vi "Algae Teleop Handler.vi"() -> ()   [LabVIEW 2023]
uses:
  Teleop Util/Algae States.ctl
  <vilib>/Rock Robotics/WPI/Joystick/XBox Buttons Indexer.ctl
  <vilib>/Rock Robotics/WPI/Joystick/XBox Axes Indexer.ctl
  Algae/Implementation/Algae Operations.ctl
  918af4a3-8dae-4537-8dc6-29252aaed449.vi
  <vilib>/Rock Robotics/WPI/Utilities/WPI_GetSetVariantRefNum.vi
  Framework/Robot Global Data.vi
panel:
  in  "Setpoint":dbl
  out "s? t:f":T1=enum."Intake Algae"
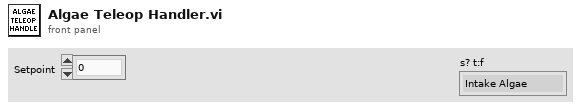
[diagram p1: front panel]
types:
  T1 = typedef "Algae States.ctl" = enum16{"Idle", "Intake Algae", "Outtake Algae", "Stow", "Manual Overrides"}
  T2 = typedef "XBox Axes Indexer.ctl" = enum16{"Left X", "Left Y", "Left Trigger", "Right Trigger", "Right X", "Right Y"}
  T3 = typedef "XBox Buttons Indexer.ctl" = enum16{"A", "B", "X", "Y", "Left Bumper", "Right Bumper", "Back", "Start", "Left Joystick", "Right Joystick"}
  T4 = typedef "WPI_JoystickDevRef.ctl" = cluster{"Device":T5}
  T5 = typedef "WPI_JoystickDeviceEnum.ctl" = enum16{"USB 0", "USB 1", "USB 2", "USB 3", "USB 4", "USB 5"}
  T6 = typedef "Algae Operations.ctl" = enum16{"Reserve", "Read Current", "Immediate", "Calibrate"}
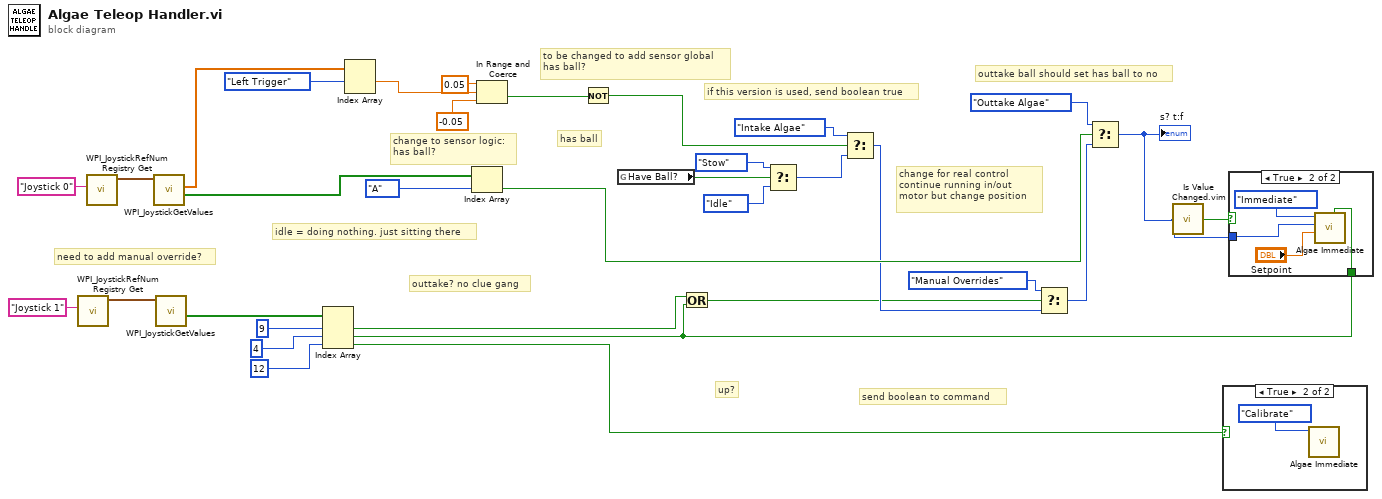
[diagram p0: block diagram]
diagram:
  # "send boolean to command"
  # "up?"
  # "if this version is used, send boolean true"
  # "outtake? no clue gang"
  # "outtake ball should set has ball to no"
  # "has ball"
  # "change for real control\ncontinue running in/out\nmotor but change position"
  # "to be changed to add sensor global\nhas ball?"
  # "need to add manual override?"
  # "idle = doing nothing. just sitting there"
  # "change to sensor logic:\nhas ball?"
  n1 = call <vilib>:"WPI_JoystickRefNum Registry Get.vi"("refnum name"="Joystick 1") -> ("JoystickDevRef"=w21:T4)  [unwired: 1 in, 9 out]
  n2 = call <vilib>:"WPI_JoystickRefNum Registry Get.vi"("refnum name"="Joystick 0") -> ("JoystickDevRef"=w32:T4)  [unwired: 1 in, 9 out]
  n3 = call <vilib>:"WPI_JoystickGetValues.vi"("JoystickDevRef"=w32) -> ("Buttons"=w31:bool[], "Axes"=w26:dbl[])  [unwired: 6 in, 3 out]
  n4 = call <vilib>:"WPI_JoystickGetValues.vi"("JoystickDevRef"=w21) -> ("Buttons"=w13:bool[])  [unwired: 6 in, 4 out]
  n5 = Index Array(array=w13, index #1=9 ("index"), index #2=4 ("index"), index #3=12 ("index")) -> (element #1=w5:bool, element #2=w4:bool, element #3=w12:bool)
  n6 = Index Array(array=w26, index #1=XBox_Axes_Indexer."Left Trigger" ("XBox Axes")) -> (element #1=w25:dbl)  [unwired: 1 in, 1 out]
  n7 = Index Array(array=w31, index=XBox_Buttons_Indexer."A" ("XBox Buttons")) -> (element=w19:bool)
  n8 = In Range and Coerce(upper limit=0.05 ("lower limit"), x=w25, lower limit=-0.05) -> (In Range?=w27:bool)  [unwired: 1 out]
  n9 = Not(x=w27) -> (.not. x?=w8:bool)
  n10 = global read "Robot Global Data.vi" "Have Ball?"() -> (w7:bool)
  n11 = Or(x=w5, y=w4) -> (x .or. y?=w6:bool)
  n12 = Select(t=Algae_States."Stow" ("f"), s=w7, f=Algae_States."Idle") -> (s? t:f=w9:T1)
  n13 = Select(t=Algae_States."Intake Algae", s=w8, f=w9) -> (s? t:f=w16:T1)
  n14 = Select(t=Algae_States."Manual Overrides", s=w6, f=w16) -> (s? t:f=w17:T1)
  n15 = Select(t=Algae_States."Outtake Algae", s=w19, f=w17) -> (s? t:f=w14:T1)
  "s? t:f" <- w14
  n16 = call "Is Value Changed.vim"("value"=w14) -> ("changed or first call?"=w15:bool)
  n17 = case shown="True" w12 {
    frame False {
    }
    frame True {
      n18 = call "Algae Immediate.vi"("Operation"=Algae_Operations."Calibrate") -> ()  [unwired: 9 in, 1 out]
    }
  }
  n19 = case shown="True" w15 {
    tunnel: w14 -> [_ w37]
    tunnel: w4 -> [_ w36]
    frame False {
    }
    frame True {
      n20 = call "Algae Immediate.vi"("Operation"=Algae_Operations."Immediate", "Algae State"=w37, "Setpoint"="Setpoint", "Negate or Confirm?"=w36) -> ()  [unwired: 6 in, 1 out]
    }
  }
